vi "Single Acquisition UI.vi"() -> ()   [LabVIEW 2014]
uses:
  <vilib>/rvi/interface/nirviOpenFPGA/nirviOpenFPGA.xnode
  <vilib>/rvi/interface/nirviMethod/nirviMethod.xnode
  <vilib>/rvi/errors/niLvFpgaMergeErrorWithErrorCode.vi
  <vilib>/FPGAPlugInAG/Dynamic/niLvFpga_Run_Dynamic.vi
  <vilib>/rvi/interface/nirviCloseFPGA/nirviCloseFPGA.xnode
  <vilib>/FPGAPlugInAG/Dynamic/niLvFpga_ConfigureFifo_Dynamic.vi
  <vilib>/FPGAPlugInAG/Dynamic/niLvFpga_StartFifo_Dynamic.vi
  <vilib>/FPGAPlugInAG/Dynamic/niLvFpga_ReadFifo_Dynamic.vi
  <vilib>/FPGAPlugInAG/Dynamic/niLvFpga_Close_Dynamic.vi
  FPGA Target/Test VIs/Acquisition Test.vi
panel:
  out "Elements Remaining":u32
  out "Waveform Graph (input data)":dbl[](graph)
  in  "Number of Elements to read":u32=512
  in  "Wave path":path
  # "This VI perform a single acquisition from the DIO."
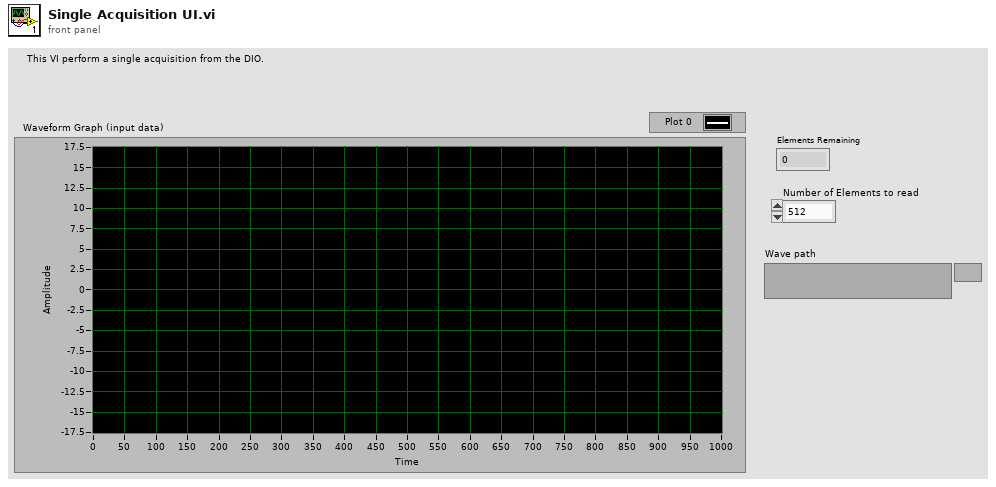
[diagram p1: front panel]
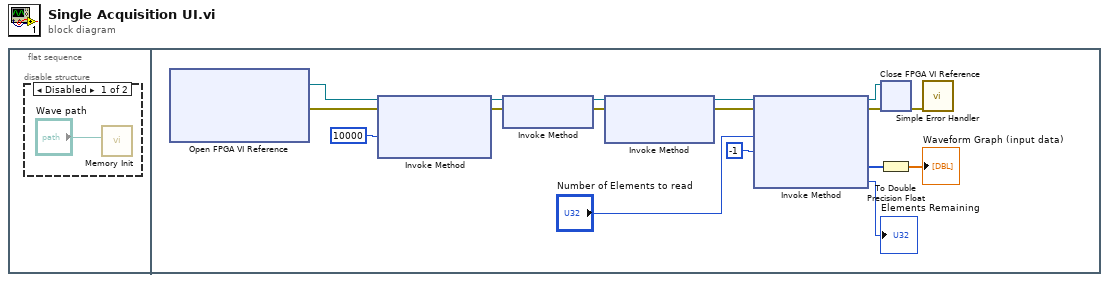
[diagram p0: block diagram]
diagram:
  n1 = flat-sequence {
    frame #0 {
      n2 = disable-structure shown="Disabled" {
        frame Disabled {
          n3 = call "Memory Init.vi"("Wave path"="Wave path") -> ()  [unwired: 9 in]
        }
        frame Enabled {
        }
      }
    }
    frame #1 {
      n4 = xnode "Open FPGA VI Reference"() -> ("FPGA VI Reference Out"=w18:refnum<k20>, "error out"=w17:errorcluster)  [unwired: 2 in]
      n5 = xnode "Invoke Method"("FPGA VI Reference In"=w18, "error in"=w17, "Requested Depth"=u32 10000) -> ("FPGA VI Reference Out"=w14:refnum<k20>, "error out"=w15:errorcluster)  [unwired: 1 out]
      n6 = xnode "Invoke Method"("FPGA VI Reference In"=w14, "error in"=w15) -> ("FPGA VI Reference Out"=w12:refnum<k20>, "error out"=w13:errorcluster)
      n7 = xnode "Invoke Method"("FPGA VI Reference In"=w12, "error in"=w13) -> ("FPGA VI Reference Out"=w11:refnum<k20>, "error out"=w10:errorcluster)  [unwired: 1 in]
      n8 = xnode "Invoke Method"("FPGA VI Reference In"=w11, "error in"=w10, "Number of Elements"="Number of Elements to read", "Timeout (ms)"=-1) -> ("FPGA VI Reference Out"=w8:refnum<k20>, "error out"=w7:errorcluster, "Data"=w3:u16[], "Elements Remaining"=→"Elements Remaining":u32)
      n9 = xnode "Close FPGA VI Reference"("FPGA VI Reference In"=w8, "error in"=w7) -> ("error out"=w9:errorcluster)
      n10 = To Double Precision Float(number=w3) -> (double precision float=→"Waveform Graph (input data)":dbl[])
      n11 = call <vilib>:"Simple Error Handler.vi"("error in (no error)"=w9) -> ()  [unwired: 4 in, 5 out]
    }
  }
